vi "Redundant Modbus Masters.vi"() -> ()   [LabVIEW 2021]
doc: "This is the launcher VI for the Redundant Modbus Masters example. This VI serves only as a window in which to view the 4 asynchronous components of the application. Each subpanel is running it's own VI which can be opened from the project explorer."
uses:
  Stop Global.vi
panel:
  in  "Stop":bool
  # "Overview: Demonstrates the implementation of redundant masters in a Modbus application.\nRequirements: LabVIEW Datalogging and Supervisory Control Module OR LabVIEW Real-Time Module\nInstructions: \n 1. Run the VI to launch all asynchronous components and loads them into subpanels.\n 2. In the Primary Modbus Master subpanel, change the Operating Mode to Simulate Crash and observe the behavior of the VI.\n 3. Right-click the border of each subpanel and click Open Block Diagram to open the block diagram of the component.\n 4. Click Stop to stop the VI."
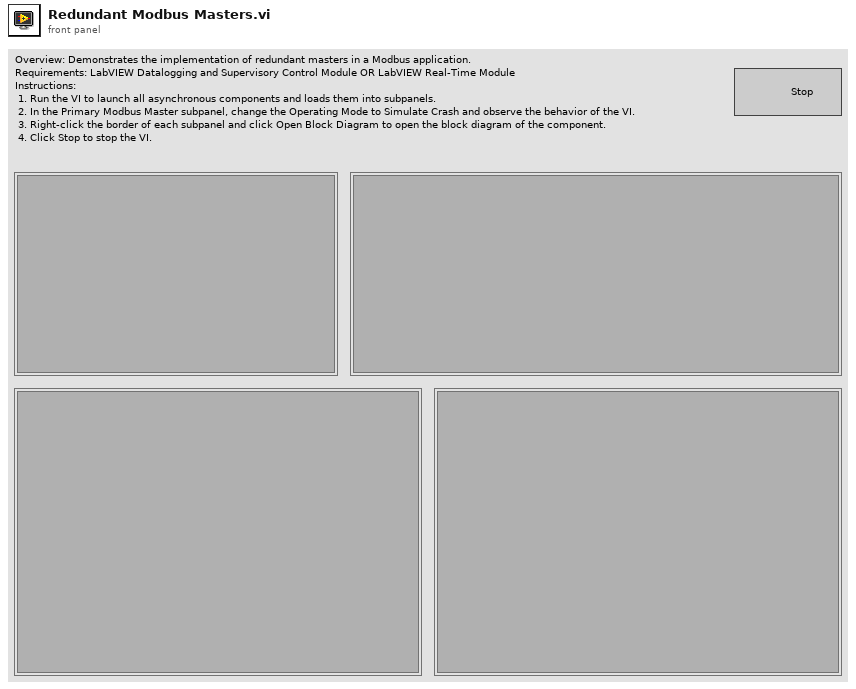
[diagram p1: front panel]
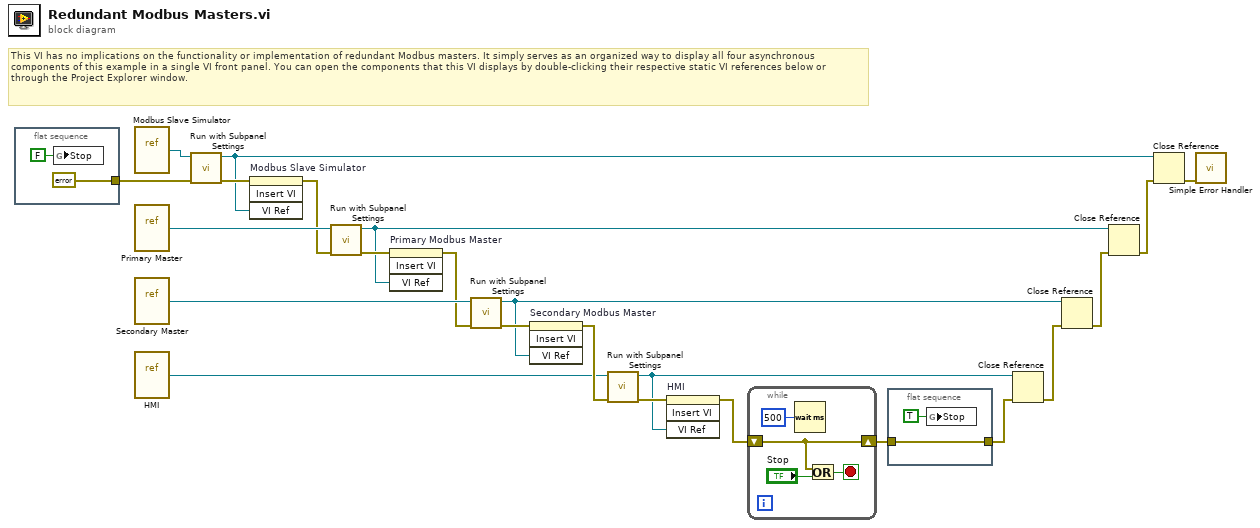
[diagram p0: block diagram]
diagram:
  # "This VI has no implications on the functionality or implementation of redundant Modbus masters. It simply serves as an organized way to display all four asynchronous components of this example in a single VI front panel. You can open the components that this VI displays by double-clicking their respective static VI references below or through the Project Explorer window."
  n1 = flat-sequence {
    tunnel: [errorcluster {"status"=FALSE, "code"=0, "source"=""} ("error constant")] -> w10
    frame #0 {
      n2 = global write "Stop Global.vi" "Stop"(FALSE ("Stop")) -> ()
    }
  }
  n3 = vi-ref "Modbus Slave Simulator.vi"() -> (w19:refnum<vi>)
  n4 = vi-ref "Primary Master.vi"() -> (w18:refnum<vi>)
  n5 = vi-ref "Secondary Master.vi"() -> (w17:refnum<vi>)
  n6 = vi-ref "HMI.vi"() -> (w11:refnum<vi>)
  n7 = call "Run with Subpanel Settings.vi"("error in (no error)"=w10, "VI Refnum In"=w19) -> ("error out"=w23:errorcluster, "VI Refnum"=w4:refnum<vi>)  [unwired: 8 in]
  n8 = invoke on="Modbus Slave Simulator" class="SubPanel" method="Insert VI"(error in=w23, "VI Ref"=w4) -> (error out=w16:errorcluster)  [unwired: 2 in, 3 out]
  n9 = call "Run with Subpanel Settings.vi"("error in (no error)"=w16, "VI Refnum In"=w18) -> ("error out"=w22:errorcluster, "VI Refnum"=w3:refnum<vi>)  [unwired: 8 in]
  n10 = invoke on="Primary Modbus Master" class="SubPnl" method="Insert VI"(error in=w22, "VI Ref"=w3) -> (error out=w15:errorcluster)  [unwired: 2 in, 3 out]
  n11 = call "Run with Subpanel Settings.vi"("error in (no error)"=w15, "VI Refnum In"=w17) -> ("error out"=w21:errorcluster, "VI Refnum"=w2:refnum<vi>)  [unwired: 8 in]
  n12 = invoke on="Secondary Modbus Master" class="SubPnl" method="Insert VI"(error in=w21, "VI Ref"=w2) -> (error out=w14:errorcluster)  [unwired: 2 in, 3 out]
  n13 = call "Run with Subpanel Settings.vi"("error in (no error)"=w14, "VI Refnum In"=w11) -> ("error out"=w20:errorcluster, "VI Refnum"=w1:refnum<vi>)  [unwired: 8 in]
  n14 = invoke on="HMI" class="SubPnl" method="Insert VI"(error in=w20, "VI Ref"=w1) -> (error out=w13:errorcluster)  [unwired: 2 in, 3 out]
  n15 = while {
    shift-right: [w27] -> w9
    shift-left: w13 -> [w27]
    stop <- w26 stop-if-true
    n16 = Wait (ms)(milliseconds to wait=u32 500) -> ()  [unwired: 1 out]
    n17 = Or(x=w27, y="Stop") -> (x .or. y?=w26:bool)
  }
  n18 = flat-sequence {
    tunnel: [w30] -> w8
    tunnel: w9 -> [w30]
    frame #0 {
      n19 = global write "Stop Global.vi" "Stop"(TRUE ("Stop")) -> ()
    }
  }
  n20 = Close Reference(reference=w1, error in (no error)=w8) -> (error out=w7:errorcluster)
  n21 = Close Reference(reference=w2, error in (no error)=w7) -> (error out=w6:errorcluster)
  n22 = Close Reference(reference=w3, error in (no error)=w6) -> (error out=w5:errorcluster)
  n23 = Close Reference(reference=w4, error in (no error)=w5) -> (error out=w12:errorcluster)
  n24 = call <vilib>:"Simple Error Handler.vi"("error in (no error)"=w12) -> ()  [unwired: 4 in, 5 out]
